vi "LVIS_VerifyConnection.vi"(8 "Error In":errorcluster) -> (0 "Error Out":errorcluster, 3 "Success?":bool)   [LabVIEW 2015]
doc: "Sends a ping request to the Data Commander IP address and throws an error if no response is received."
uses:
  Ctrls/LVIS_SAF Status.ctl
  Globals/LVIS_DcGlobals.vi
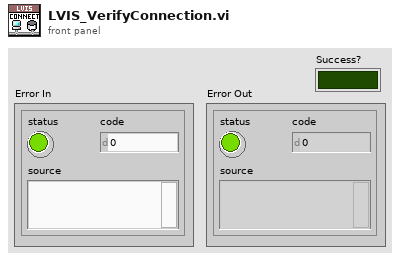
[diagram p1: front panel]
types:
  T1 = cluster{"DCIP":string, "BackupFile":string, "ErrorLog":string, "FilePosition":string}
  T2 = typedef "LVIS_SAF Status.ctl" = u16
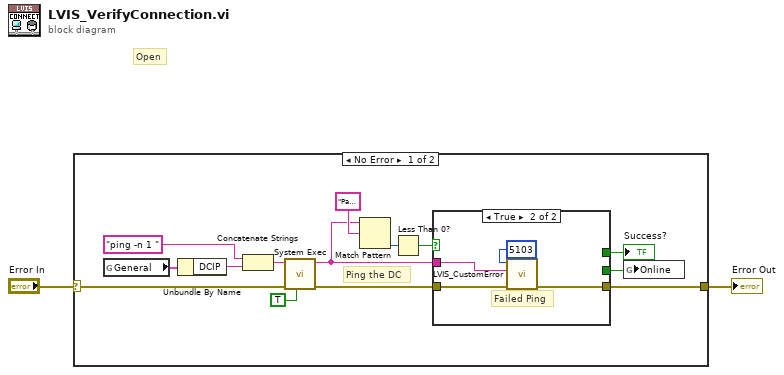
[diagram p0: block diagram]
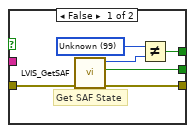
[diagram p2: hidden frame]
diagram:
  # "Open"
  n1 = case shown="No Error" "Error In" {
    selector: "Error In" -> [w16 w27]
    tunnel: [w6 w27] -> w2
    frame No Error {
      # "Ping the DC"
      n2 = global read "LVIS_DcGlobals.vi" "General"() -> (w14:T1)
      n3 = Unbundle By Name(w14) -> ("DCIP"=w13:string)
      n4 = Concatenate Strings("ping -n 1 ", w13) -> (w12:string)
      n5 = call <vilib>:"System Exec.vi"("run minimized? (F)"=TRUE, "error in (no error)"=w16, "command line"=w12) -> ("error out"=w8:errorcluster, "standard output"=w7:string)  [unwired: 5 in, 2 out]
      n6 = Match Pattern(string=w7, regular expression="Packets: Sent = 1, Received = 1, Lost = 0") -> (offset past match=w9:i32)  [unwired: 1 in, 3 out]
      n7 = Less Than 0?(x=w9) -> (x < 0?=w3:bool)
      n8 = case shown="True" w3 {
        tunnel: w8 -> [w22 w25]
        tunnel: w7 -> [_ w23]
        tunnel: [w18 w24] -> w6
        tunnel: [w19 _] -> w5
        tunnel: [w17 _] -> w4
        frame False {
          w20 = T2 99 items=["Clear"=0, "SAF Active"=100, "SAF Complete"=101, "SAF > 50%"=102, "SAF < 50%"=103, "SAF Full"=104, "Unknown"=99] ("x")
          # "Get SAF State"
          n9 = call "LVIS_GetSAF.vi"("Error In"=w22) -> ("Error out"=w18:errorcluster, "Online?"=w17:bool, "SAF State"=w21:T2)  [unwired: 8 in]
          n10 = Not Equal?(x=w20, y=w21) -> (x != y?=w19:bool)
        }
        frame True {
          # "Failed Ping"
          n11 = call "LVIS_CustomError.vi"("error in (no error)"=w25, "Addiitional Info"=w23, "Code"=5103) -> ("error out"=w24:errorcluster)  [unwired: 8 in]
        }
      }
      "Success?" <- w5
      n12 = global write "LVIS_DcGlobals.vi" "Online"(w4) -> ()
    }
    frame Error {
    }
  }
  "Error Out" <- w2
